vi "5.10 Recording Buffers.vi"() -> (0 "Recording Buffers":T1)   [LabVIEW 2010]
uses:
  5.10 Buffers Cluster.ctl
  <vilib>/userDefined/High Color/IMAQdx.ctl
  <vilib>/vision/Image Controls.llb/IMAQ Image.ctl
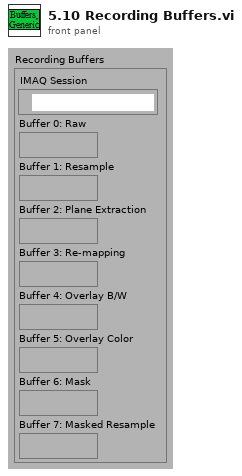
[diagram p1: front panel]
types:
  T1 = typedef "5.10 Buffers Cluster.ctl" = cluster{"IMAQ Session":T2, "Buffer 0: Raw":T3, "Buffer 1: Resample":T3, "Buffer 2: Plane Extraction":T3, "Buffer 3: Re-mapping":T3, "Buffer 4: Overlay B/W":T3, "Buffer 5: Overlay Color":T3, "Buffer 6: Mask":T3, "Buffer 7: Masked Resample":T3}
  T2 = typedef "IMAQdx.ctl" = refnum<k21>
  T3 = typedef "IMAQ Image.ctl" = refnum<image>
  T4 = typedef "Image Type" = u32
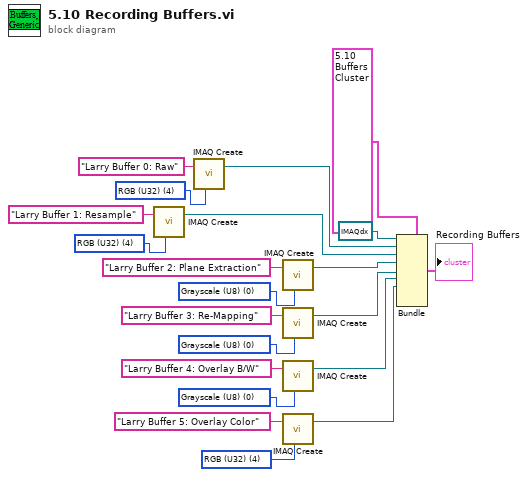
[diagram p0: block diagram]
diagram:
  w13 = T4 4 items=["Grayscale (U8)", "Grayscale (I16)", "Grayscale (SGL)", "Complex (CSG)", "RGB (U32)", "HSL (U32)", "RGB (U64)", "Grayscale (U16)"] ("Image Type")
  w10 = T4 0 items=["Grayscale (U8)", "Grayscale (I16)", "Grayscale (SGL)", "Complex (CSG)", "RGB (U32)", "HSL (U32)", "RGB (U64)", "Grayscale (U16)"] ("Image Type")
  w9 = T4 4 items=["Grayscale (U8)", "Grayscale (I16)", "Grayscale (SGL)", "Complex (CSG)", "RGB (U32)", "HSL (U32)", "RGB (U64)", "Grayscale (U16)"] ("Image Type")
  w6 = T4 4 items=["Grayscale (U8)", "Grayscale (I16)", "Grayscale (SGL)", "Complex (CSG)", "RGB (U32)", "HSL (U32)", "RGB (U64)", "Grayscale (U16)"] ("Image Type")
  w5 = T4 0 items=["Grayscale (U8)", "Grayscale (I16)", "Grayscale (SGL)", "Complex (CSG)", "RGB (U32)", "HSL (U32)", "RGB (U64)", "Grayscale (U16)"] ("Image Type")
  w2 = T4 0 items=["Grayscale (U8)", "Grayscale (I16)", "Grayscale (SGL)", "Complex (CSG)", "RGB (U32)", "HSL (U32)", "RGB (U64)", "Grayscale (U16)"] ("Image Type")
  n1 = call "IMAQ Create"("Image Name"="Larry Buffer 1: Resample", "Image Type"=w9) -> ("New Image"=w15:T3)  [unwired: 3 in, 1 out]
  n2 = call "IMAQ Create"("Image Name"="Larry Buffer 0: Raw", "Image Type"=w13) -> ("New Image"=w14:T3)  [unwired: 3 in, 1 out]
  n3 = call "IMAQ Create"("Image Name"="Larry Buffer 2: Plane Extraction", "Image Type"=w10) -> ("New Image"=w16:T3)  [unwired: 3 in, 1 out]
  n4 = call "IMAQ Create"("Image Name"="Larry Buffer 3: Re-Mapping", "Image Type"=w5) -> ("New Image"=w17:T3)  [unwired: 3 in, 1 out]
  n5 = call "IMAQ Create"("Image Name"="Larry Buffer 4: Overlay B/W", "Image Type"=w2) -> ("New Image"=w18:T3)  [unwired: 3 in, 1 out]
  n6 = call "IMAQ Create"("Image Name"="Larry Buffer 5: Overlay Color", "Image Type"=w6) -> ("New Image"=w19:T3)  [unwired: 3 in, 1 out]
  n7 = Bundle(cluster=T1 {"IMAQ Session"="", "Buffer 0: Raw"=refnum, "Buffer 1: Resample"=refnum, "Buffer 2: Plane Extraction"=refnum, "Buffer 3: Re-mapping"=refnum, "Buffer 4: Overlay B/W"=refnum, "Buffer 5: Overlay Color"=refnum, "Buffer 6: Mask"=refnum, "Buffer 7: Masked Resample"=refnum} ("output cluster"), "IMAQ Session"=T2 refnum, "Buffer 0: Raw"=w14, "Buffer 1: Resample"=w15, "Buffer 2: Plane Extraction"=w16, "Buffer 3: Re-mapping"=w17, "Buffer 4: Overlay B/W"=w18, "Buffer 5: Overlay Color"=w19) -> (→"Recording Buffers":T1)  [unwired: 2 in]
